vi "Configure Serial Input DMA FIFOs.vi"(0 "fpga interface in":refnum<k20>, 5 "serial channels":string[](array[string]), 7 "llp data dma fifo depth (elements)":u32=10240000, 11 "error in (no error)":errorcluster) -> (4 "fpga interface out":refnum<k20>, 15 "error out":errorcluster)   [LabVIEW 2023, in "GettingStarted_Acq_148X_Host.lvlib"]
uses:
  GettingStarted_Acq_148X_Host.lvlib
  Types/148x_Acq_FPGA_Reference.ctl
  <vilib>/rvi/interface/common/niFpgaWaitOnOcc.vi
  <vilib>/rvi/interface/nirviMethod/nirviMethod.xnode
  <vilib>/rvi/errors/niLvFpgaMergeErrorWithErrorCode.vi
  <vilib>/FPGAPlugInAG/Dynamic/niLvFpga_ConfigureFifo_Dynamic.vi
  <vilib>/FPGAPlugInAG/Dynamic/niLvFpga_StartFifo_Dynamic.vi
  <instrlib>/FlexRIO/Automotive Vision Utility/v1/Host/Automotive Vision Utility.lvlib
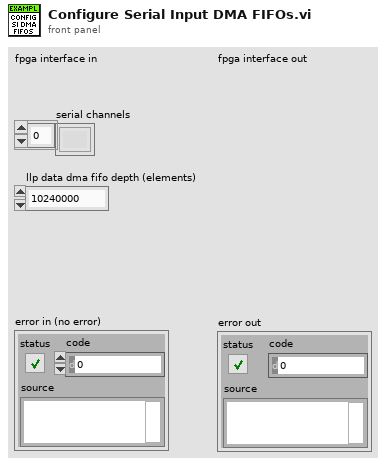
[diagram p1: front panel]
types:
  T1 = typedef "GettingStarted_Acq_148X_Host.lvlib/148x_Acq_FPGA_Reference.ctl" = refnum<k20>
  T2 = typedef "Automotive Vision Utility.lvlib/Serial Channel Type.ctl" = enum16{"Serial Input Channel", "Serial Output Channel", "Unknown Channel Type"}
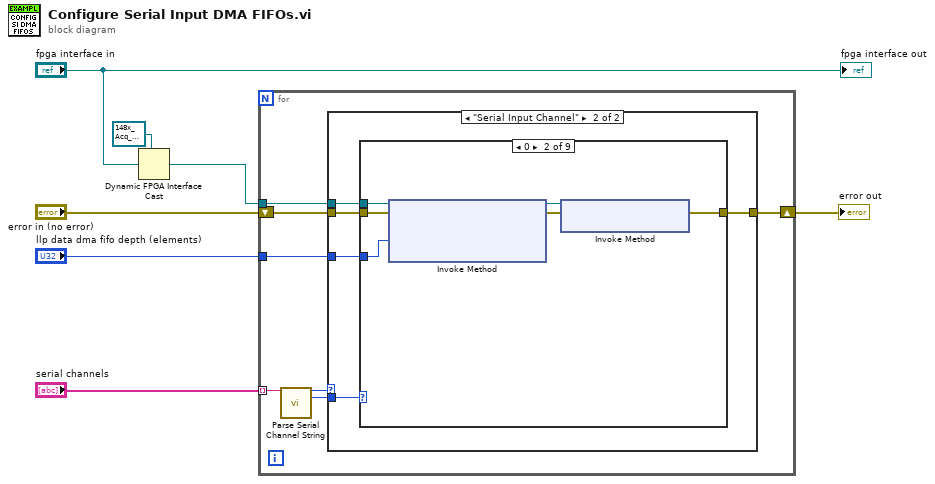
[diagram p0: block diagram]
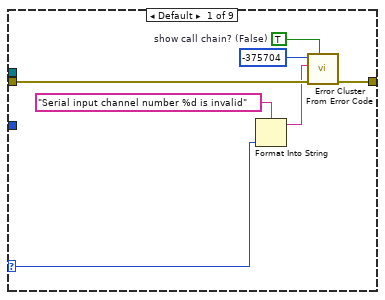
[diagram p3: hidden frame]
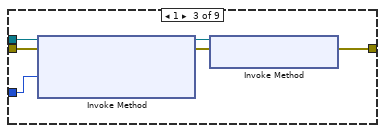
[diagram p4: hidden frame]
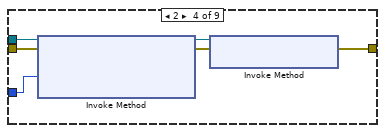
[diagram p5: hidden frame]
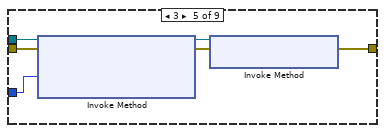
[diagram p6: hidden frame]
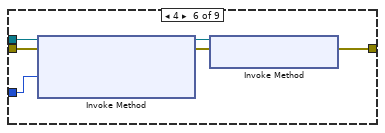
[diagram p7: hidden frame]
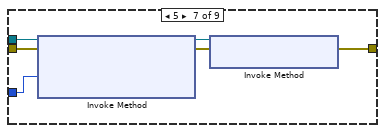
[diagram p8: hidden frame]
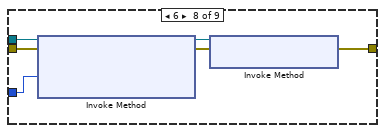
[diagram p9: hidden frame]
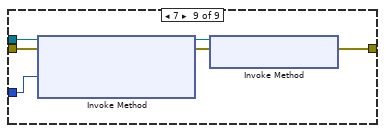
[diagram p10: hidden frame]
diagram:
  n1 = Dynamic FPGA Interface Cast(Session In=T1 refnum ("FPGA VI Reference Out"), Type="fpga interface in") -> (Session Out=w4:T1)
  n2 = for {
    tunnel: "llp data dma fifo depth (elements)" -> [w13]
    tunnel: w4 -> [w12]
    shift-right: [w11] -> w2
    shift-left: "error in (no error)" -> [w14]
    tunnel: "serial channels" -> [w10] mode=indexing
    n3 = call <instrlib>:"Parse Serial Channel String.vi"("serial channel string"=w10) -> ("serial channel type"=w9:T2, "channel number"=w8:i32)  [unwired: 13 in]
    n4 = case shown="\"Serial Input Channel\"" w9 {
      tunnel: w14 -> [w15 w20]
      tunnel: w13 -> [_ w19]
      tunnel: w12 -> [_ w18]
      tunnel: [w15 w17] -> w11
      tunnel: w8 -> [_ w16]
      frame Default {
      }
      frame "Serial Input Channel" {
        n5 = case shown="0" w16 {
          selector: w16 -> [w21 _ _ _ _ _ _ _ _]
          tunnel: w20 -> [w24 w31 w37 w43 w49 w55 w61 w67 w73]
          tunnel: w19 -> [_ w29 w34 w40 w47 w52 w58 w64 w70]
          tunnel: w18 -> [_ w30 w36 w42 w48 w54 w60 w66 w72]
          tunnel: [w25 w28 w35 w41 w46 w53 w59 w65 w71] -> w17
          frame Default {
            w26 = TRUE  # show call chain? (False)
            n6 = Format Into String(format string="Serial input channel number %d is invalid" ("error message (\"\")"), w21) -> (resulting string=w22:string)  [unwired: 2 in, 1 out]
            n7 = call <vilib>:"Error Cluster From Error Code.vi"("show call chain? (False)"=w26, "error in (no error)"=w24, "error message (\"\")"=w22, "error code (0)"=-375704) -> ("error out"=w25:errorcluster)  [unwired: 5 in]
          }
          frame 0 {
            n8 = xnode "Invoke Method"("FPGA VI Reference In"=w30, "error in"=w31, "Requested Depth"=w29) -> ("FPGA VI Reference Out"=w32:T1, "error out"=w33:errorcluster)  [unwired: 1 out]
            n9 = xnode "Invoke Method"("FPGA VI Reference In"=w32, "error in"=w33) -> ("error out"=w28:errorcluster)  [unwired: 1 out]
          }
          frame 1 {
            n10 = xnode "Invoke Method"("FPGA VI Reference In"=w36, "error in"=w37, "Requested Depth"=w34) -> ("FPGA VI Reference Out"=w38:T1, "error out"=w39:errorcluster)  [unwired: 1 out]
            n11 = xnode "Invoke Method"("FPGA VI Reference In"=w38, "error in"=w39) -> ("error out"=w35:errorcluster)  [unwired: 1 out]
          }
          frame 2 {
            n12 = xnode "Invoke Method"("FPGA VI Reference In"=w42, "error in"=w43, "Requested Depth"=w40) -> ("FPGA VI Reference Out"=w44:T1, "error out"=w45:errorcluster)  [unwired: 1 out]
            n13 = xnode "Invoke Method"("FPGA VI Reference In"=w44, "error in"=w45) -> ("error out"=w41:errorcluster)  [unwired: 1 out]
          }
          frame 3 {
            n14 = xnode "Invoke Method"("FPGA VI Reference In"=w48, "error in"=w49, "Requested Depth"=w47) -> ("FPGA VI Reference Out"=w50:T1, "error out"=w51:errorcluster)  [unwired: 1 out]
            n15 = xnode "Invoke Method"("FPGA VI Reference In"=w50, "error in"=w51) -> ("error out"=w46:errorcluster)  [unwired: 1 out]
          }
          frame 4 {
            n16 = xnode "Invoke Method"("FPGA VI Reference In"=w54, "error in"=w55, "Requested Depth"=w52) -> ("FPGA VI Reference Out"=w56:T1, "error out"=w57:errorcluster)  [unwired: 1 out]
            n17 = xnode "Invoke Method"("FPGA VI Reference In"=w56, "error in"=w57) -> ("error out"=w53:errorcluster)  [unwired: 1 out]
          }
          frame 5 {
            n18 = xnode "Invoke Method"("FPGA VI Reference In"=w60, "error in"=w61, "Requested Depth"=w58) -> ("FPGA VI Reference Out"=w62:T1, "error out"=w63:errorcluster)  [unwired: 1 out]
            n19 = xnode "Invoke Method"("FPGA VI Reference In"=w62, "error in"=w63) -> ("error out"=w59:errorcluster)  [unwired: 1 out]
          }
          frame 6 {
            n20 = xnode "Invoke Method"("FPGA VI Reference In"=w66, "error in"=w67, "Requested Depth"=w64) -> ("FPGA VI Reference Out"=w68:T1, "error out"=w69:errorcluster)  [unwired: 1 out]
            n21 = xnode "Invoke Method"("FPGA VI Reference In"=w68, "error in"=w69) -> ("error out"=w65:errorcluster)  [unwired: 1 out]
          }
          frame 7 {
            n22 = xnode "Invoke Method"("FPGA VI Reference In"=w72, "error in"=w73, "Requested Depth"=w70) -> ("FPGA VI Reference Out"=w74:T1, "error out"=w75:errorcluster)  [unwired: 1 out]
            n23 = xnode "Invoke Method"("FPGA VI Reference In"=w74, "error in"=w75) -> ("error out"=w71:errorcluster)  [unwired: 1 out]
          }
        }
      }
    }
  }
  "error out" <- w2
  "fpga interface out" <- "fpga interface in"
